vi "find readout time.vi"(8 "error in (no error)":errorcluster, 11 "Simulated_CCD_Camera in":refnum<class "Simulated_CCD_Camera.lvclass">) -> (0 "error out":errorcluster, 2 "readout time":dbl, 3 "Simulated_CCD_Camera out":refnum<class "Simulated_CCD_Camera.lvclass">)   [LabVIEW 2018, in "Simulated_CCD_Camera.lvclass"]
doc: "Find the readout time as a function of the operation mode of the CCD.\n\nThis value is used to determine the minimum exposure time allowed by ACS, that is the readout time plus 10 % of this value. This procedure is related to the functioning of the frame transfer mode of the CCD and it prevents the misuse of the exposure time."
uses:
  Simulated_CCD_Camera.lvclass
  Simulated_CCD_Camera.lvclass/Simulated_CCD_Camera.ctl
  <vilib>/Utility/file.llb/Read Delimited Spreadsheet (DBL).vi
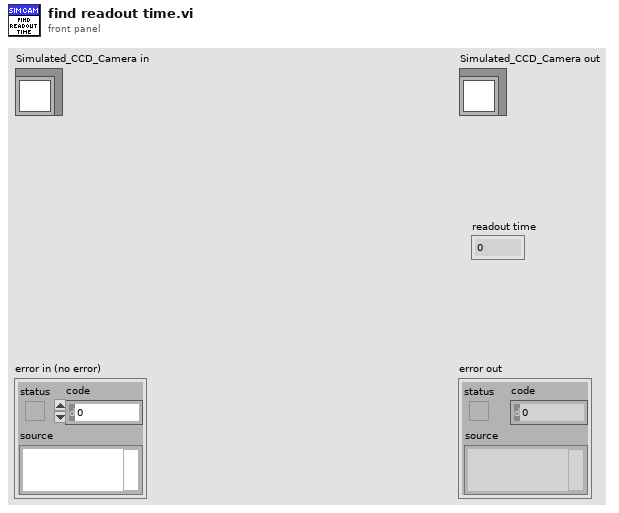
[diagram p1: front panel]
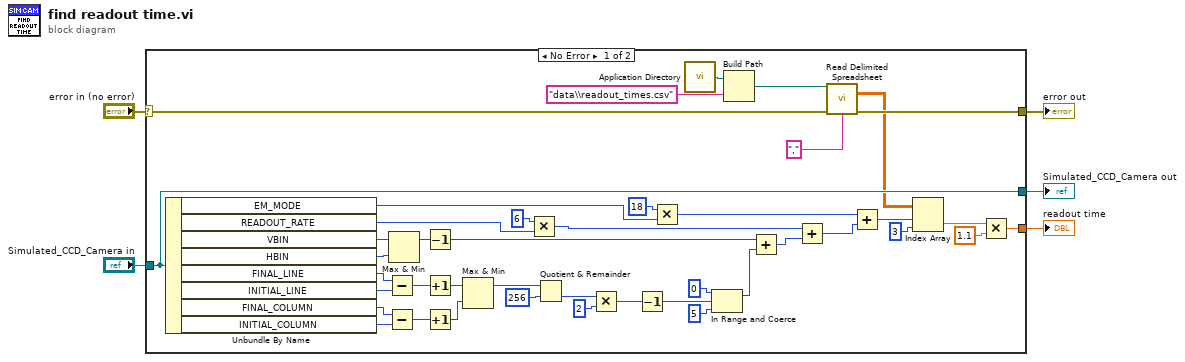
[diagram p0: block diagram]
diagram:
  n1 = case shown="No Error" "error in (no error)" {
    selector: "error in (no error)" -> [w47 w49]
    tunnel: [w46 w49] -> w4
    tunnel: [w35 w48] -> w2
    tunnel: "Simulated_CCD_Camera in" -> [w35 w48]
    tunnel: [w7 _] -> w1
    frame No Error {
      n2 = Unbundle By Name(w35) -> ("EM_MODE"=w22:u16, "READOUT_RATE"=w26:u16, "VBIN"=w30:u16, "HBIN"=w29:u16, "FINAL_LINE"=w39:u16, "INITIAL_LINE"=w38:u16, "FINAL_COLUMN"=w37:u16, "INITIAL_COLUMN"=w36:u16)
      n3 = Subtract(x=w39, y=w38) -> (x-y=w41:u16)
      n4 = Subtract(x=w37, y=w36) -> (x-y=w40:u16)
      n5 = Max & Min(x=w30, y=w29) -> (max(x,y)=w28:u16)  [unwired: 1 out]
      n6 = Decrement(x=w28) -> (x-1=w27:u16)
      n7 = Increment(x=w41) -> (x+1=w34:u16)
      n8 = Increment(x=w40) -> (x+1=w33:u16)
      n9 = Max & Min(x=w34, y=w33) -> (max(x,y)=w31:u16)  [unwired: 1 out]
      n10 = Multiply(x=u16 6, y=w26) -> (x*y=w23:u16)
      n11 = Quotient & Remainder(x=w31, y=u16 256) -> (floor(x/y)=w13:u16)  [unwired: 1 out]
      n12 = Multiply(x=w13, y=u16 2 ("x")) -> (x*y=w14:u16)
      n13 = Decrement(x=w14) -> (x-1=w12:u16)
      n14 = Multiply(x=u16 18, y=w22) -> (x*y=w19:u16)
      n15 = call <vilib>:"Application Directory.vi"() -> ("Application Directory"=w42:path)
      n16 = In Range and Coerce(upper limit=u16 0, x=w12, lower limit=u16 5 ("upper limit")) -> (coerced(x)=w9:u16)  [unwired: 1 out]
      n17 = Build Path(base path=w42, name or relative path="data\\readout_times.csv" ("delimiter (\\t)")) -> (appended path=w44:path)
      n18 = Add(x=w27, y=w9) -> (x+y=w24:u16)
      n19 = Add(x=w23, y=w24) -> (x+y=w20:u16)
      n20 = call-poly <vilib>:"Read Delimited Spreadsheet.vi"("file path (dialog if empty)"=w44, "error in (no error)"=w47, "delimiter (\\t)"="," ("delimiter (\\t)")) -> ("all rows"=w18:dbl[][], "error out"=w46:errorcluster)  [unwired: 7 in, 4 out]
      n21 = Add(x=w19, y=w20) -> (x+y=w16:u16)
      n22 = Index Array(array=w18, index (row)=w16, index (col)=3 ("disabled index (col)")) -> (element=w8:dbl)
      n23 = Multiply(x=w8, y=1.1) -> (x*y=w7:dbl)
    }
    frame Error {
    }
  }
  "error out" <- w4
  "Simulated_CCD_Camera out" <- w2
  "readout time" <- w1
